vi "Standalone REST via Automagic ControlRef Endpoints.vi"() -> ()   [LabVIEW 2023]
uses:
  Log/Log_Level.ctl
  API Message/API Message.lvclass
  Server/Control Ref Endpoint Access Mode.ctl
  Log/Log_Facilities.ctl
  Response/Standard Response Messages.ctl
  baea4f90-ed66-40c9-855f-b5689293d002.vi
  baea4f90-ed66-40c9-855f-b5689293d002.vi/bf0030c7-b76b-4182-9f9e-16cd2e366061.vi
  Request/Get Request.vi
  Response/Set Body.vi
  Response/Set Content Type.vi
  Response/Set Status Code.vi
  Response/Send.vi
  <vilib>/Platform/browser.llb/Open URL in Default Browser (string).vi
  Request/Request.lvclass
  Response/Response.lvclass
  Log/Log.lvclass
  Server/Server.lvclass
panel:
  in  "Test 2":bool
  in  "Read 1":bool
  in  "Thing 2":string="Value 2"
  in  "Thing 1":string="Value 1"
  in  "stop":bool
  # "These buttons simply open the system defaul browser to \nGET the value from the REST endpoints for these 2 strings"
  # "These endpoints would normally consumed by another\nprogram, not a browser."
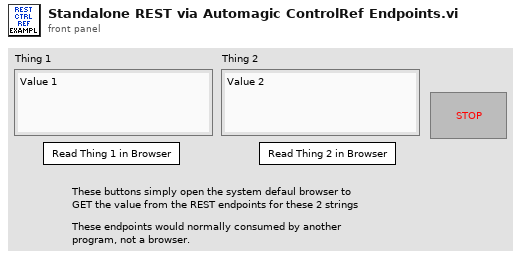
[diagram p1: front panel]
types:
  T1 = typedef "Server.lvclass/Control Ref Endpoint Access Mode.ctl" = enum16{"None", "Read/Write", "Read Only", "Write Only"}
  T2 = typedef "Log.lvclass/Log_Level.ctl" = enum16{"none", "info", "trace", "warn", "error", "fatal"}
  T3 = enum32{"invalid app kind", "Development System", "Run Time System", "Student Edition", "Embedded LabVIEW", "Evaluation", "Custom"}
  T4 = typedef "Log.lvclass/Log_Facilities.ctl" = string
  T5 = typedef "Request.ctl" = cluster{"Method":string, "URI":string, "Protocol":string, "Raw Path":string, "Query":string, "Fragment":string, "Raw Body":string, "Headers":variant, "Parameters":variant, "Body":variant, "Raw Header":string, "Path":string[]}
  T6 = typedef "Response.lvclass/Standard Response Messages.ctl" = u16
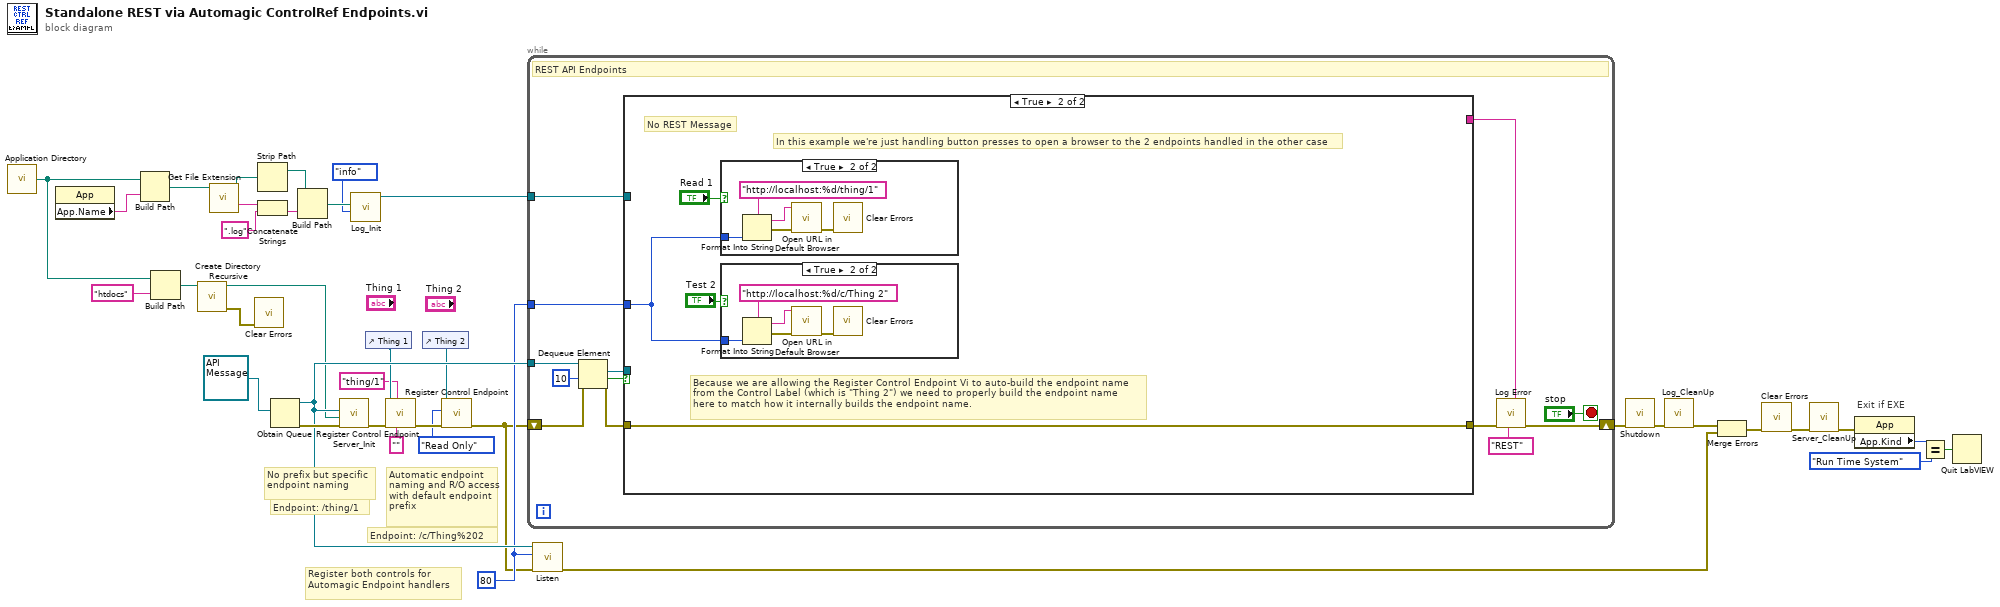
[diagram p0: block diagram]
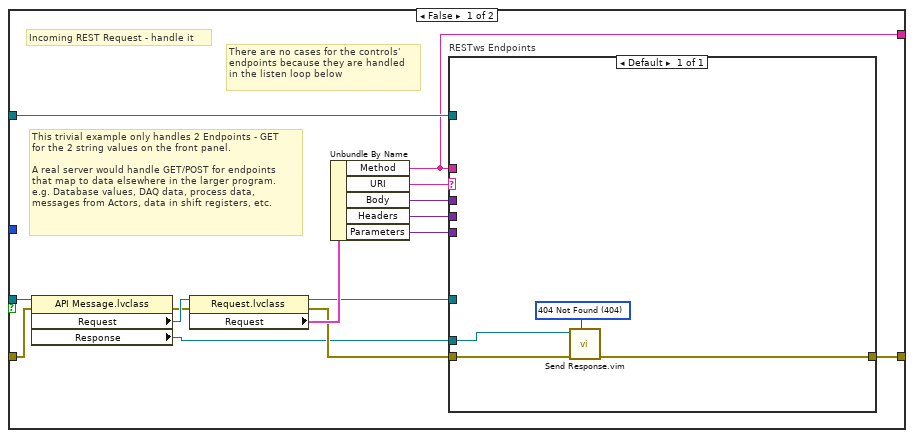
[diagram p2: hidden frame]
diagram:
  w12 = u16 80 ("Listen Port (80)")
  # "Endpoint: /c/Thing%202"
  # "Endpoint: /thing/1"
  # "Automatic endpoint naming and R/O access with default endpoint prefix"
  # "No prefix but specific endpoint naming"
  # "Register both controls for Automagic Endpoint handlers"
  # "Exit if EXE"
  n1 = call <vilib>:"Application Directory.vi"() -> ("Application Directory"=w25:path)
  n2 = property class="App"() -> ("App.Name"=w21:string)  [unwired: 2 in, 2 out]
  n3 = Build Path(base path=w25, name or relative path=w21) -> (appended path=w22:path)
  n4 = Build Path(base path=w25, name or relative path="htdocs" ("section")) -> (appended path=w11:path)
  n5 = call <vilib>:"Create Directory Recursive.vi"("directory"=w11) -> ("error out"=w9:errorcluster, "directory copy"=w10:path)  [unwired: 4 in, 1 out]
  n6 = call <vilib>:"Get File Extension.vi"("file"=w22) -> ("filename without extension"=w30:string, "dup file"=w29:path)  [unwired: 6 in, 3 out]
  n7 = call <vilib>:"Clear Errors.vi"("error in (no error)"=w9) -> ()  [unwired: 5 in, 2 out]
  n8 = Strip Path(path=w29) -> (stripped path=w28:path)  [unwired: 1 out]
  n9 = Concatenate Strings(w30, ".log" ("section")) -> (w33:string)
  n10 = Obtain Queue(element data type=refnum<class "API Message.lvclass"> refnum ("API Message.lvclass")) -> (queue out=w23:refnum<queue>, error out=w27:errorcluster)  [unwired: 4 in, 1 out]
  n11 = Build Path(base path=w28, name or relative path=w33) -> (appended path=w32:path)
  n12 = call "Server_Init.vi"("error in (no error)"=w27, "Static Data Folder"=w10, "API Queue"=w23) -> ("error out"=w8:errorcluster)  [unwired: 7 in, 1 out]
  n13 = call "Log_Init.vi"("Level"=Log_Level."info", "Log File"=w32) -> ("reference out"=w18:refnum<class "Log.lvclass">)  [unwired: 8 in, 1 out]
  n14 = control-ref of="Thing 1"() -> (w6:refnum<vi>)
  n15 = call "Register Control Endpoint.vi"("Endpoint Prefix (\"/c\")"="", "Endpoint Name (\"\"=Use Control Label)"="thing/1", "Error In"=w8, "Control Ref"=w6) -> ("Error Out"=w7:errorcluster)  [unwired: 7 in]
  n16 = control-ref of="Thing 2"() -> (w5:refnum<vi>)
  n17 = call "Register Control Endpoint.vi"("Error In"=w7, "Endpoint Access Mode (Read/Write)"=Control_Ref_Endpoint_Access_Mode."Read Only", "Control Ref"=w5) -> ("Error Out"=w1:errorcluster)  [unwired: 8 in]
  n18 = while "Send to RT" {
    shift-right: [w41] -> w16
    shift-left: w1 -> [w45]
    tunnel: w23 -> [w50]
    tunnel: w18 -> [w43]
    tunnel: w12 -> [w38]
    stop <- "stop" stop-if-true
    # "REST API Endpoints"
    n19 = Dequeue Element(queue=w50, timeout in ms (-1)=10, error in (no error)=w45) -> (element=w47:refnum<class "API Message.lvclass">, timed out?=w49:bool, error out=w48:errorcluster)  [unwired: 1 out]
    n20 = case shown="True" w49 {
      tunnel: w48 -> [w64 w73]
      tunnel: [w58 w73] -> w42
      tunnel: w47 -> [w65 _]
      tunnel: w43 -> [w54 _]
      tunnel: [w53 _] -> w39
      tunnel: w38 -> [_ w70]
      frame False {
        # "There are no cases for the controls'\nendpoints because they are handled\nin the listen loop below"
        # "This trivial example only handles 2 Endpoints - GET\nfor the 2 string values on the front panel.\n\nA real server would handle GET/POST for endpoints\nthat map to data elsewhere in the larger program.\ne.g. Database values, DAQ data, process data, \nmessages from Actors, data in shift registers, etc."
        # "Incoming REST Request - handle it"
        n21 = property class="API Message.lvclass"(reference=w65, error in=w64) -> (error out=w62:errorcluster, "Request"=w63:refnum<class "Request.lvclass">, "Response"=w56:refnum<class "Response.lvclass">)  [unwired: 1 out]
        n22 = property class="Request.lvclass"(reference=w63, error in=w62) -> (reference out=w57:refnum<class "Request.lvclass">, error out=w59:errorcluster, "Request"=w61:T5)
        n23 = Unbundle By Name(w61) -> ("Method"=w53:string, "URI"=w60:string, "Body"=w55:variant, "Headers"=w52:variant, "Parameters"=w51:variant)
        n24 = case "RESTws Endpoints" shown="Default" w60 {
          tunnel: w59 -> [w68]
          tunnel: [w69] -> w58
          tunnel: w53 -> [_]
          tunnel: w57 -> [_]
          tunnel: w56 -> [w67]
          tunnel: w55 -> [_]
          tunnel: w54 -> [_]
          tunnel: w52 -> [_]
          tunnel: w51 -> [_]
          frame Default {
            w66 = T6 404 items=["200 OK"=200, "201 Created"=201, "202 Accepted"=202, "203 Non-Authoritative Information"=203, "204 No Content"=204, "205 Reset Content"=205, "206 Partial Content"=206, "207 Multi-Status (WebDAV)"=207, "208 Already Reported (WebDAV)"=208, "226 IM Used (HTTP Delta encoding)"=226, "300 Multiple Choices"=300, "301 Moved Permanently"=301, "302 Found"=302, "303 See Other"=303, "304 Not Modified"=304, "305 Use Proxy Deprecated"=305, "307 Temporary Redirect"=307, "308 Permanent Redirect"=308, "400 Bad Request"=400, "401 Unauthorized"=401, "402 Payment Required"=402, "403 Forbidden"=403, "404 Not Found"=404, "405 Method Not Allowed"=405, "406 Not Acceptable"=406, "407 Proxy Authentication Required"=407, "408 Request Timeout"=408, "409 Conflict"=409, "410 Gone"=410, "411 Length Required"=411, "412 Precondition Failed"=412, "413 Content Too Large"=413, "414 URI Too Long"=414, "415 Unsupported Media Type"=415, "416 Range Not Satisfiable"=416, "417 Expectation Failed"=417, "418 I'm a teapot"=418, "421 Misdirected Request"=421, "422 Unprocessable Content (WebDAV)"=422, "423 Locked (WebDAV)"=423, "424 Failed Dependency (WebDAV)"=424, "425 Too Early Experimental"=425, "426 Upgrade Required"=426, "428 Precondition Required"=428, "429 Too Many Requests"=429, "431 Request Header Fields Too Large"=431, "451 Unavailable For Legal Reasons"=451, "500 Internal Server Error"=500, "501 Not Implemented"=501, "502 Bad Gateway"=502, "503 Service Unavailable"=503, "504 Gateway Timeout"=504, "505 HTTP Version Not Supported"=505, "506 Variant Also Negotiates"=506, "507 Insufficient Storage (WebDAV)"=507, "508 Loop Detected (WebDAV)"=508, "510 Not Extended"=510, "511 Network Authentication Required"=511] ("Status Codes")
            n25 = call "Send Response.vim"("Status Code (200=OK)"=w66, "Error In"=w68, "Response"=w67) -> ("Error Out"=w69:errorcluster)  [unwired: 8 in]
          }
        }
      }
      frame True {
        # "Because we are allowing the Register Control Endpoint Vi to auto-build the endpoint name\nfrom the Control Label (which is \"Thing 2\") we need to properly build the endpoint name\nhere to match how it internally builds the endpoint name."
        # "In this example we're just handling button presses to open a browser to the 2 endpoints handled in the other case"
        # "No REST Message"
        n26 = case shown="True" "Read 1" {
          tunnel: w70 -> [_ w83]
          frame False {
          }
          frame True {
            n27 = Format Into String(format string="http://localhost:%d/thing/1", w83) -> (resulting string=w79:string, error out=w81:errorcluster)  [unwired: 2 in]
            n28 = call-poly <vilib>:"Open URL in Default Browser.vi"("error in (no error)"=w81, "URL"=w79) -> ("error out"=w80:errorcluster)  [unwired: 4 in, 1 out]
            n29 = call <vilib>:"Clear Errors.vi"("error in (no error)"=w80) -> ()  [unwired: 5 in, 2 out]
          }
        }
        n30 = case shown="True" "Test 2" {
          tunnel: w70 -> [_ w78]
          frame False {
          }
          frame True {
            n31 = Format Into String(format string="http://localhost:%d/c/Thing 2", w78) -> (resulting string=w74:string, error out=w76:errorcluster)  [unwired: 2 in]
            n32 = call-poly <vilib>:"Open URL in Default Browser.vi"("error in (no error)"=w76, "URL"=w74) -> ("error out"=w75:errorcluster)  [unwired: 4 in, 1 out]
            n33 = call <vilib>:"Clear Errors.vi"("error in (no error)"=w75) -> ()  [unwired: 5 in, 2 out]
          }
        }
      }
    }
    n34 = call "Log Error.vi"("Context"=w39, "Facility (default)"=T4 "REST", "error in (no error)"=w42) -> ("error out"=w41:errorcluster)  [unwired: 8 in]
  }
  n35 = call "Listen.vi"("error in (no error)"=w1, "Listen Port (80)"=w12, "API Queue"=w23) -> ("error out"=w19:errorcluster)  [unwired: 8 in]
  n36 = call "Shutdown.vi"("error in (no error)"=w16) -> ("error out"=w15:errorcluster)  [unwired: 10 in]
  n37 = call "Log_CleanUp.vi"("error in (no error)"=w15) -> ("error out"=w17:errorcluster)  [unwired: 10 in]
  n38 = Merge Errors(w17, w19) -> (w20:errorcluster)
  n39 = call <vilib>:"Clear Errors.vi"("error in (no error)"=w20) -> ("error out"=w14:errorcluster)  [unwired: 5 in, 1 out]
  n40 = call "Server_CleanUp.vi"("error in (no error)"=w14) -> ("error out"=w13:errorcluster)  [unwired: 10 in]
  n41 = property class="App"(error in=w13) -> ("App.Kind"=w37:T3)  [unwired: 1 in, 2 out]
  n42 = Equal?(x=w37, y=T3."Run Time System" ("Application:Kind")) -> (x = y?=w35:bool)
  n43 = Quit LabVIEW(quit? (T)=w35) -> ()
